vi "to_json.vi"(8 "error in":errorcluster, 11 "noManifest in":refnum<class "noManifest.lvclass">) -> (0 "error out":errorcluster, 2 "json":string, 3 "noManifest out":refnum<class "noManifest.lvclass">, 4 "Not Default":bool)   [LabVIEW 2020, in "nominal types.lvlib" / "timestampManifest.lvlib" / "noManifest.lvclass"]
uses:
  noManifest.lvclass
  noManifest.lvclass/noManifest.ctl
  3ea01a1e-9b4b-4b52-9ce8-3c2677203621.vi
  startingTimestamp.get.vi
  scaleParameter.get.vi
  <vilib>/JDP Science/JSONtext/Variant to JSON Text.vi
  <vilib>/JDP Science/JSONtext/support/Format JSON Object.vi
  scaleParameter/scaleParameter.lvclass
  <vilib>/JDP Science/JSONtext/LVClass Serializer/JSONtext LVClass Serializer.lvclass
  <vilib>/JDP Science/JSONtext/JSONtext.lvlib
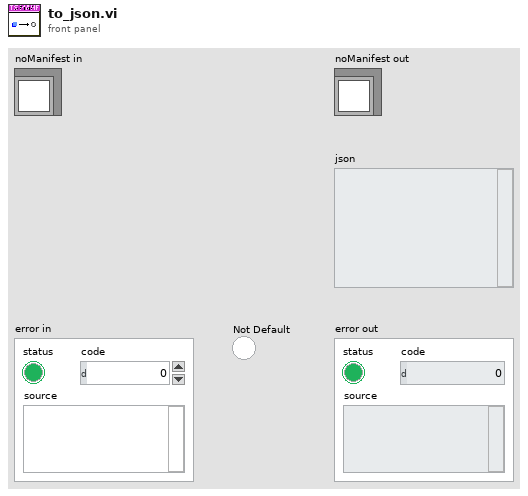
[diagram p1: front panel]
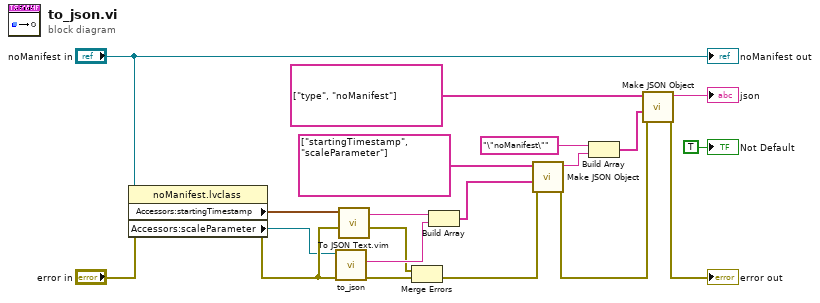
[diagram p0: block diagram]
diagram:
  n1 = property class="noManifest.lvclass"(reference="noManifest in", error in="error in") -> (error out=w8:errorcluster, "Accessors:startingTimestamp"=w20:cluster{"seconds":i64, "nanos":i64, "picos":i64}, "Accessors:scaleParameter"=w1:refnum<class "scaleParameter.lvclass">)  [unwired: 1 out]
  n2 = call-dynamic "to_json.vi"("error in"=w8, "scaleParameter in"=w1) -> ("error out"=w6:errorcluster, "json"=w17:string)  [unwired: 6 in, 2 out]
  n3 = call "To JSON Text.vim"("error in (no error)"=w8, "Anything"=w20) -> ("error out"=w7:errorcluster, "<JSON>"=w18:string)  [unwired: 8 in]
  n4 = Merge Errors(w7, w6) -> (w5:errorcluster)
  n5 = Build Array(w18, w17) -> (w16:string[])
  n6 = call <vilib>:"Make JSON Object.vi"("error in (no error)"=w5, "JSON Items"=w16, "Item Names"=string[] ["startingTimestamp", "scaleParameter"]) -> ("error out"=w4:errorcluster, "<JSON>"=w14:string)  [unwired: 7 in]
  n7 = Build Array("\"noManifest\"" ("String"), w14) -> (w13:string[])
  n8 = call <vilib>:"Make JSON Object.vi"("error in (no error)"=w4, "JSON Items"=w13, "Item Names"=string[] ["type", "noManifest"]) -> ("error out"=→"error out":errorcluster, "<JSON>"=→"json":string)  [unwired: 7 in]
  "noManifest out" <- "noManifest in"
  "Not Default" <- TRUE ("Not Default")
